vi "Shift_007.vi"() -> ()   [LabVIEW 2019]
panel:
  out "Energies":dbl[unit][][](array[numeric])
  out "Eenrgies":dbl[unit][][](graph)
  in  "time threshold 2":dbl[unit]=5.0
  in  "Control Force 2":dbl[unit]=1000.0
  in  "time threshold 1":dbl[unit]=2.0
  in  "Control Force 1":dbl[unit]=1000.0
  in  "D":dbl[unit]=25.0
  out "Ep(tk)":dbl[unit][](array[numeric])
  out "Et(tk)":dbl[unit][](array[numeric])
  out "Ek(tk)":dbl[unit][](array[numeric])
  out "Et":cluster{dbl[unit][], dbl[unit][]}(graph)
  out "Ep":cluster{dbl[unit][], dbl[unit][]}(graph)
  out "Ek":cluster{dbl[unit][], dbl[unit][]}(graph)
  out "Et":dbl[unit][](graph)
  out "Ep":dbl[unit][](graph)
  out "Ek":dbl[unit][](graph)
  out "a":cluster{dbl[unit][], dbl[unit][]}(graph)
  out "v":cluster{dbl[unit][], dbl[unit][]}(graph)
  out "x":cluster{dbl[unit][], dbl[unit][]}(graph)
  out "time (tk)":dbl[unit][](array[numeric])
  out "a":dbl[unit][](graph)
  out "v":dbl[unit][](graph)
  out "x":dbl[unit][](graph)
  out "x(tk)":dbl[unit][](array[numeric])
  out "v(tk)":dbl[unit][](array[numeric])
  out "a(tk)":dbl[unit][](array[numeric])
  in  "M":dbl[unit]=100.0
  in  "k":dbl[unit]=1000.0
  in  "v0":dbl[unit]
  in  "x0":dbl[unit]=2.0
  in  "Dt":dbl[unit]=1e-05
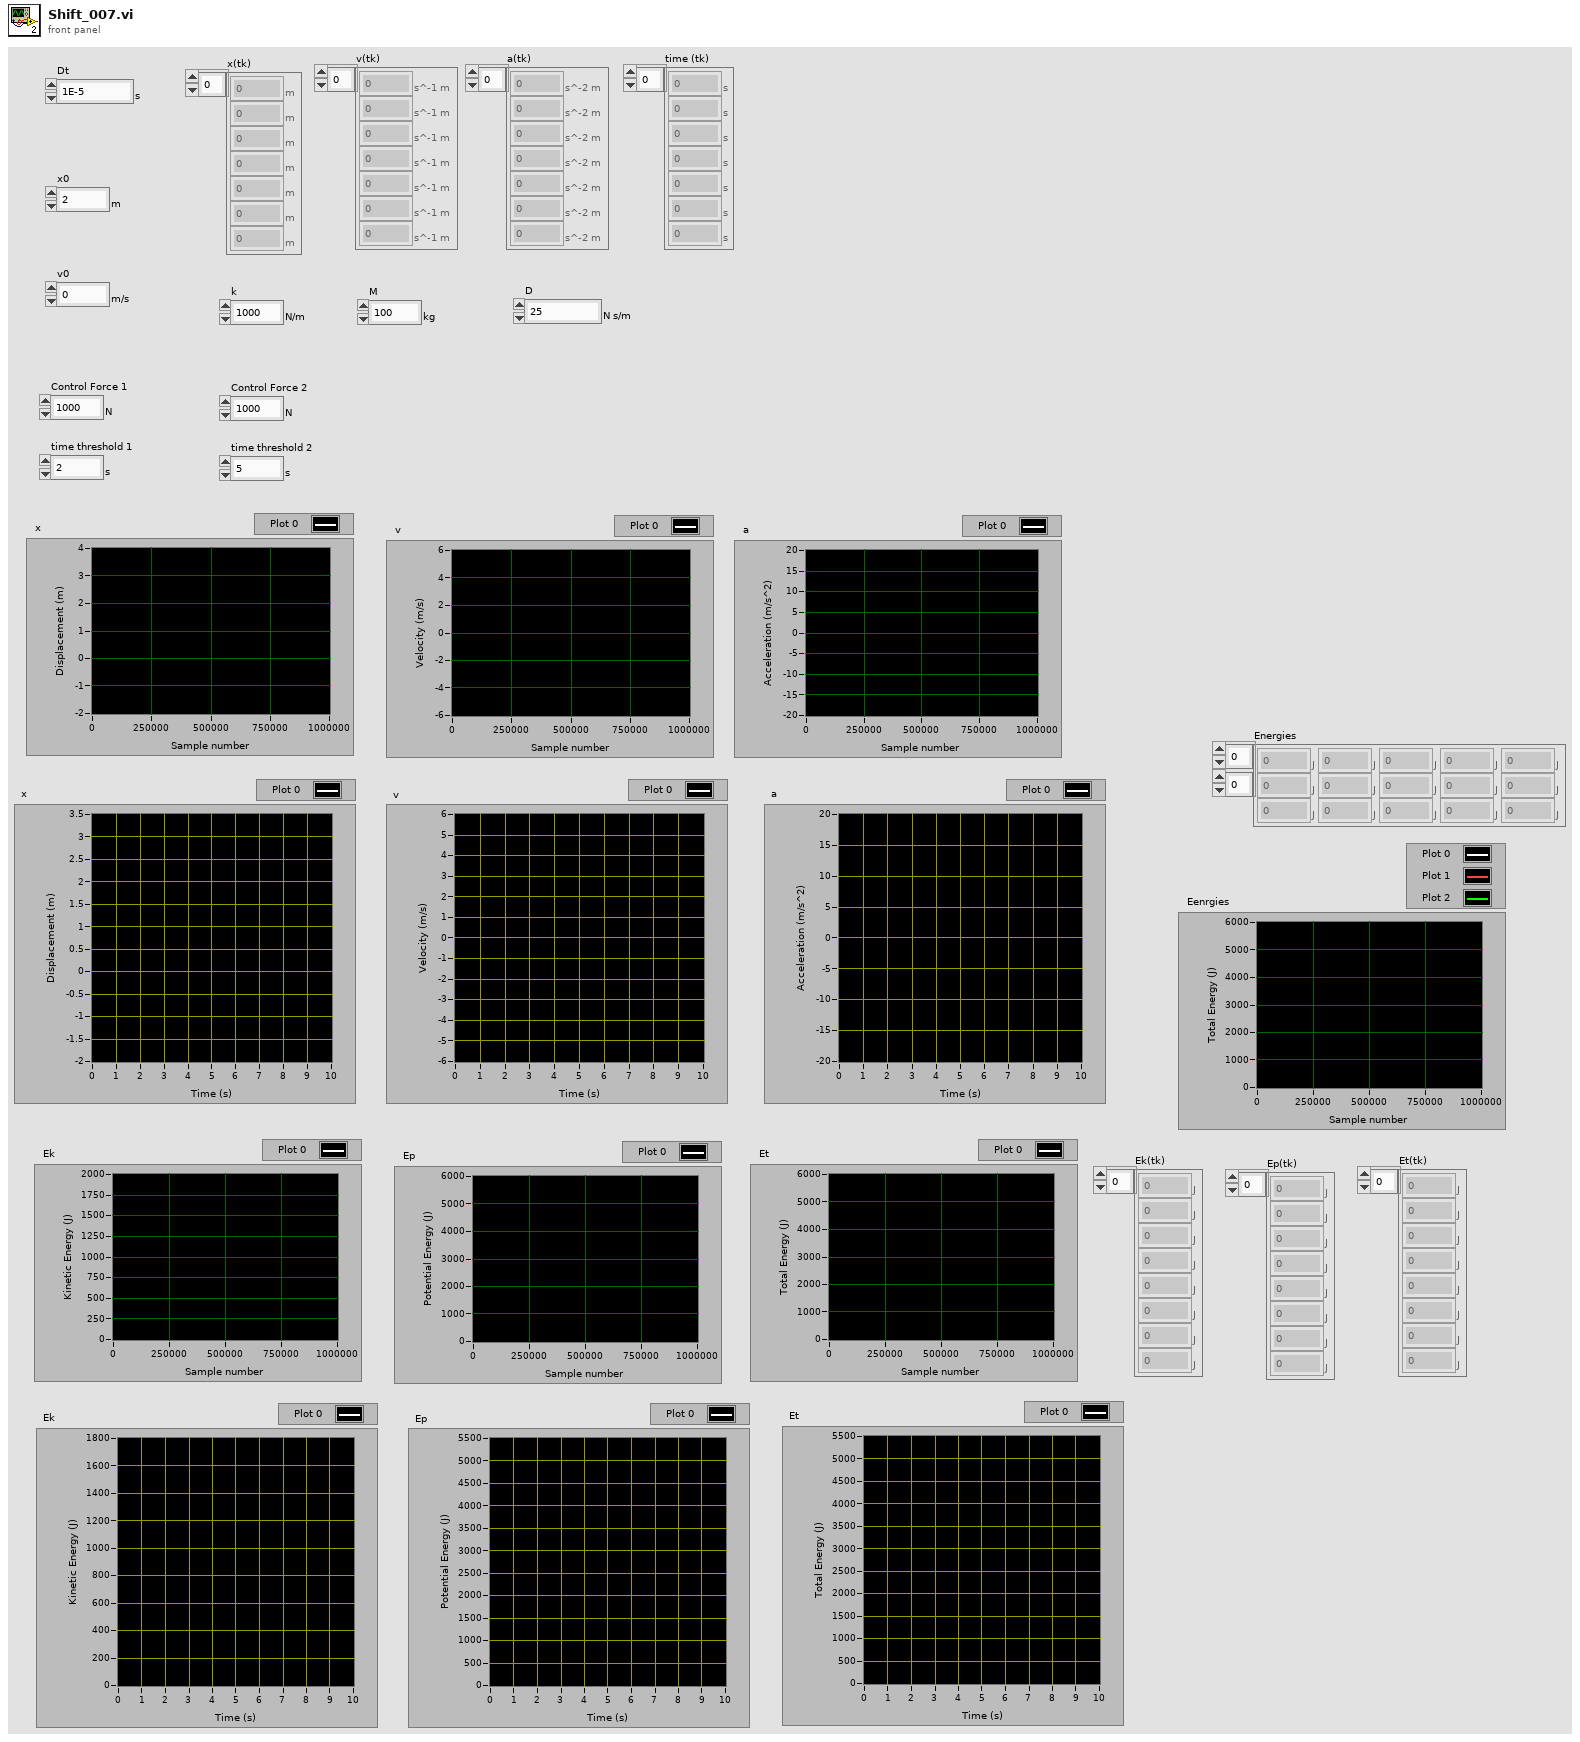
[diagram p1: front panel]
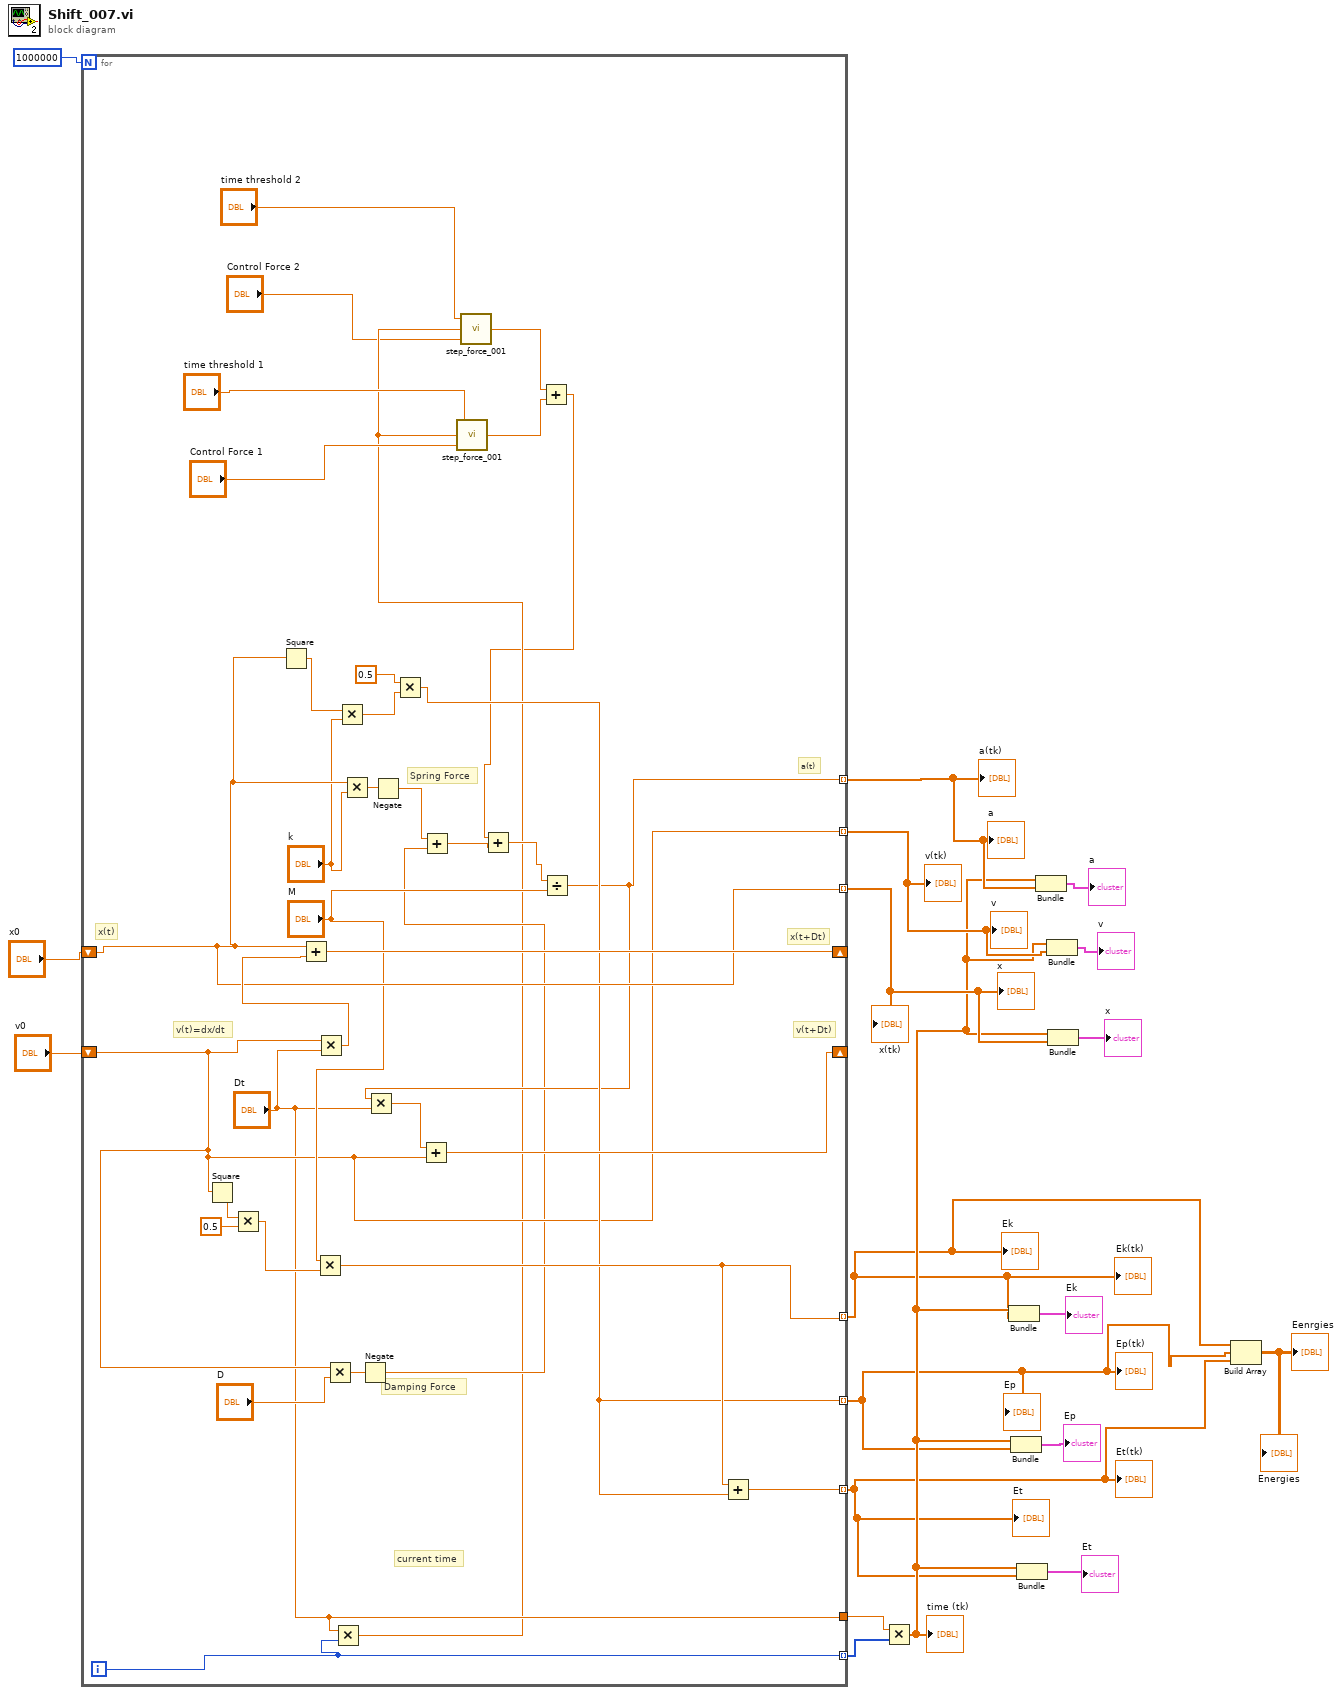
[diagram p0: block diagram]
diagram:
  n1 = for {
    N: 1000000 -> [_]
    shift-right: [w53] -> _
    shift-left: "x0" -> [w47]
    shift-right: [w50] -> _
    shift-left: "v0" -> [w37]
    tunnel: [w33] -> w11 mode=indexing
    tunnel: [w37] -> w10 mode=indexing
    tunnel: [w47] -> w9 mode=indexing
    tunnel: [w28] -> w15 mode=indexing
    tunnel: ["Dt"] -> w16
    tunnel: [w42] -> w4 mode=indexing
    tunnel: [w39] -> w3 mode=indexing
    tunnel: [w41] -> w2 mode=indexing
    i -> [w28]
    # "current time"
    # "Spring Force"
    # "Damping Force"
    # "a(t)"
    # "v(t+Dt)"
    # "x(t+Dt)"
    # "v(t)=dx/dt"
    # "x(t)"
    n2 = Square(x=w37) -> (x^2=w48:dbl[unit])
    n3 = Multiply(x=w48, y=0.5) -> (x*y=w43:dbl[unit])
    n4 = Square(x=w47) -> (x^2=w46:dbl[unit])
    n5 = Multiply(x="M", y=w43) -> (x*y=w42:dbl[unit])
    n6 = Multiply(x=w37, y="Dt") -> (x*y=w54:dbl[unit])
    n7 = Add(x=w47, y=w54) -> (x+y=w53:dbl[unit])
    n8 = Multiply(x=w37, y="D") -> (x*y=w36:dbl[unit])
    n9 = Multiply(x="Dt", y=w28) -> (x*y=w25:dbl[unit])
    n10 = Multiply(x=w46, y="k") -> (x*y=w45:dbl[unit])
    n11 = Multiply(x=w47, y="k") -> (x*y=w52:dbl[unit])
    n12 = Negate(x=w36) -> (-x=w32:dbl[unit])
    n13 = Negate(x=w52) -> (-x=w34:dbl[unit])
    n14 = Multiply(x=0.5, y=w45) -> (x*y=w39:dbl[unit])
    n15 = Add(x=w34, y=w32) -> (x+y=w31:dbl[unit])
    n16 = call "step_force_001.vi"("Control Force in"="Control Force 1", "Current time"=w25, "time threshold"="time threshold 1") -> ("Control Force out"=w22:dbl[unit])
    n17 = call "step_force_001.vi"("Control Force in"="Control Force 2", "Current time"=w25, "time threshold"="time threshold 2") -> ("Control Force out"=w21:dbl[unit])
    n18 = Add(x=w21, y=w22) -> (x+y=w20:dbl[unit])
    n19 = Add(x=w20, y=w31) -> (x+y=w30:dbl[unit])
    n20 = Divide(x=w30, y="M") -> (x/y=w33:dbl[unit])
    n21 = Multiply(x=w33, y="Dt") -> (x*y=w51:dbl[unit])
    n22 = Add(x=w51, y=w37) -> (x+y=w50:dbl[unit])
    n23 = Add(x=w42, y=w39) -> (x+y=w41:dbl[unit])
  }
  "a(tk)" <- w11
  "v(tk)" <- w10
  "x(tk)" <- w9
  "v" <- w10
  "a" <- w11
  "x" <- w9
  "Et" <- w2
  "Ek" <- w4
  "Ep" <- w3
  "Ek(tk)" <- w4
  "Et(tk)" <- w2
  "Ep(tk)" <- w3
  n24 = Multiply(x=w16, y=w15) -> (x*y=w5:dbl[unit][])
  "time (tk)" <- w5
  n25 = Bundle(w5, w4) -> (→"Ek":cluster{dbl[unit][], dbl[unit][]})  [unwired: 1 in]
  n26 = Bundle(w5, w3) -> (→"Ep":cluster{dbl[unit][], dbl[unit][]})  [unwired: 1 in]
  n27 = Bundle(w5, w2) -> (→"Et":cluster{dbl[unit][], dbl[unit][]})  [unwired: 1 in]
  n28 = Bundle(w5, w11) -> (→"a":cluster{dbl[unit][], dbl[unit][]})  [unwired: 1 in]
  n29 = Bundle(w5, w10) -> (→"v":cluster{dbl[unit][], dbl[unit][]})  [unwired: 1 in]
  n30 = Bundle(w5, w9) -> (→"x":cluster{dbl[unit][], dbl[unit][]})  [unwired: 1 in]
  n31 = Build Array(w4, w3, w2) -> (→"Eenrgies" →"Energies":dbl[unit][][])
